vi "Release Queue.vi"(8 "error in (no error)":errorcluster, 11 "LVQueue Sink in":refnum<class "LVQueue Sink.lvclass">) -> (0 "error out":errorcluster, 3 "Remaining Elements":T1[](array[typedef]))   [LabVIEW 2019, in "LVQueue Sink.lvclass"]
uses:
  <vilib>/gpm_packages/@cs/event-logger/Source/LVQueue Sink/LVQueue Sink.lvclass
  <vilib>/gpm_packages/@cs/event-logger/Source/Composed Log/Types/Log Packet.ctl
  <vilib>/gpm_packages/@cs/event-logger/Source/Composed Log/Types/Log Level.ctl
  <vilib>/gpm_packages/@cs/event-logger/Source/LVQueue Sink/LVQueue Sink.lvclass/LVQueue Sink.ctl
  <vilib>/gpm_packages/@cs/event-logger/Source/Composed Log/Composed Log.lvlib
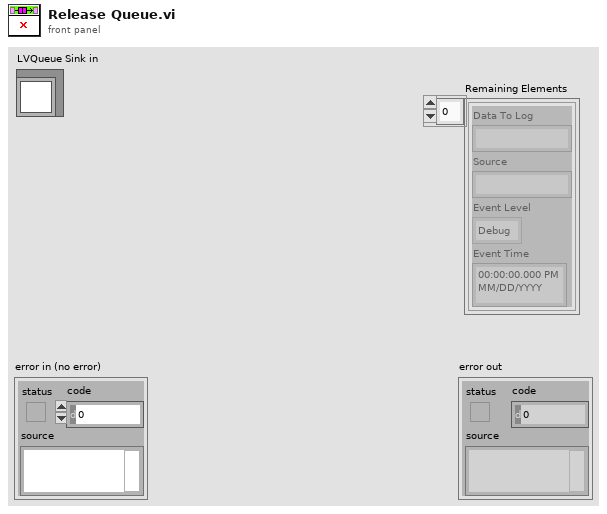
[diagram p1: front panel]
types:
  T1 = typedef "Composed Log.lvlib/Log Packet.ctl" = cluster{"Data To Log":string, "Source":string, "Event Level":T2, "Event Time":timestamp}
  T2 = typedef "Composed Log.lvlib/Log Level.ctl" = enum16{"Debug", "Info", "Warning", "Error", "Critical"}
  T3 = typedef "Composed Log.lvlib/Application Logger.lvclass/Log Packet.ctl" = cluster{"Data To Log":string, "Source":string, "Event Level":T4, "Event Time":timestamp}
  T4 = typedef "Composed Log.lvlib/Log Sink.lvclass/Log Level.ctl" = enum16{"Debug", "Info", "Warning", "Error", "Critical"}
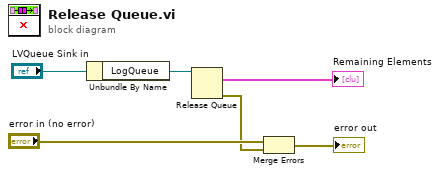
[diagram p0: block diagram]
diagram:
  n1 = Unbundle By Name("LVQueue Sink in") -> ("LogQueue"=w6:refnum<queue>)
  n2 = Release Queue(queue=w6) -> (remaining elements=→"Remaining Elements":T3[], error out=w3:errorcluster)  [unwired: 2 in, 1 out]
  n3 = Merge Errors("error in (no error)", w3) -> (→"error out":errorcluster)
